vi "Read Timestamp.vi"(8 "error in (no error)":errorcluster, 11 "DataPoint in":refnum<class "DataPoint.lvclass">) -> (0 "error out":errorcluster, 2 "Timestamp":timestamp format="%<%I:%M:%S%3u %p\n%Y/%m/%d>T", 3 "DataPoint out":refnum<class "DataPoint.lvclass">)   [LabVIEW 2018, in "InfluxDB Client.lvlib" / "DataPoint.lvclass"]
uses:
  DataPoint.lvclass
  DataPoint.lvclass/DataPoint.ctl
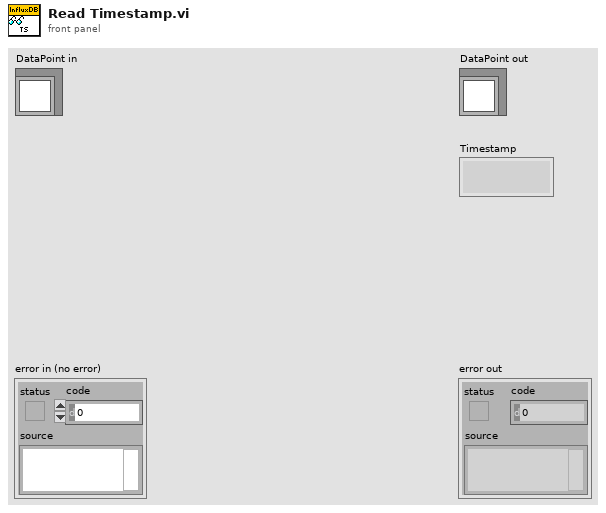
[diagram p1: front panel]
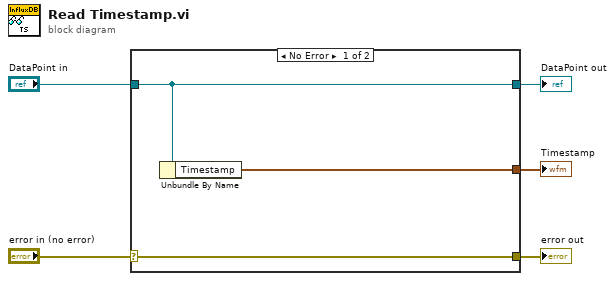
[diagram p0: block diagram]
diagram:
  n1 = case shown="No Error" "error in (no error)" {
    selector: "error in (no error)" -> [w8 w9]
    tunnel: [w8 w9] -> w4
    tunnel: [w7 w10] -> w2
    tunnel: "DataPoint in" -> [w7 w10]
    tunnel: [w6 _] -> w1
    frame No Error {
      n2 = Unbundle By Name(w7) -> ("Timestamp"=w6:timestamp)
    }
    frame Error {
    }
  }
  "error out" <- w4
  "DataPoint out" <- w2
  "Timestamp" <- w1
